vi "remove from memory format.vi"(8 "error in":errorcluster, 10 "CEF_serializable configuration in":refnum<class "CEF_serializable configuration.lvclass">, 11 "memory hierarchy in":T1) -> (0 "error out":errorcluster, 3 "memory hierarchy out":T1)   [LabVIEW 2025, in "CEF.lvlib"]
doc: "Removes an object from an object hierarchy, along with all children.Copyright 2017 National Instruments Corporation\n\nLicensed under the Apache License, Version 2.0 (the \"License\"); you may not use this file except in compliance with the License. You may obtain a copy of the License at http://www.apache.org/licenses/LICENSE-2.0\nUnless required by applicable law or agreed to in writing, software distributed under the License is distributed on an \"AS IS\" BASIS, WITHOUT WARRANTIES OR CONDITIONS OF ANY KIND, either express or implied. See the License for the specific language governing permissions and limitations under the License."
uses:
  CEF.lvlib
  hierarchy repo/memory hierarchy.ctl
  hierarchy repo/full hierarchy.ctl
  hierarchy element.ctl
  serializable configuration/CEF_serializable configuration.lvclass
  serializable configuration/CEF_serializable configuration.lvclass/CEF_serializable configuration.ctl
  <vilib>/Utility/LVClass/Get LV Class Name.vi
  error generator/CEF_error generator.vi
  hierarchy repo/CEF_HierarchyRepo.lvclass
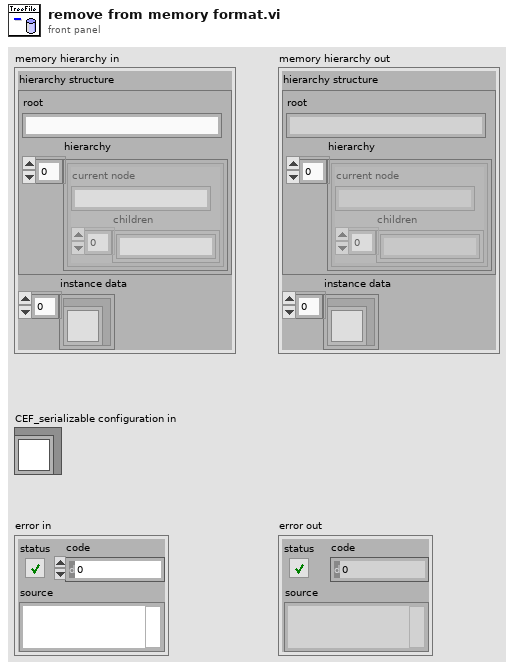
[diagram p1: front panel]
types:
  T1 = typedef "CEF.lvlib/CEF_HierarchyRepo.lvclass/memory hierarchy.ctl" = cluster{"hierarchy structure":T2, "instance data":refnum<class "CEF_serializable configuration.lvclass">[]}
  T2 = typedef "CEF.lvlib/CEF_HierarchyRepo.lvclass/full hierarchy.ctl" = cluster{"root":string, "hierarchy":T3[]}
  T3 = typedef "CEF.lvlib/hierarchy element.ctl" = cluster{"current node":string, "children":string[]}
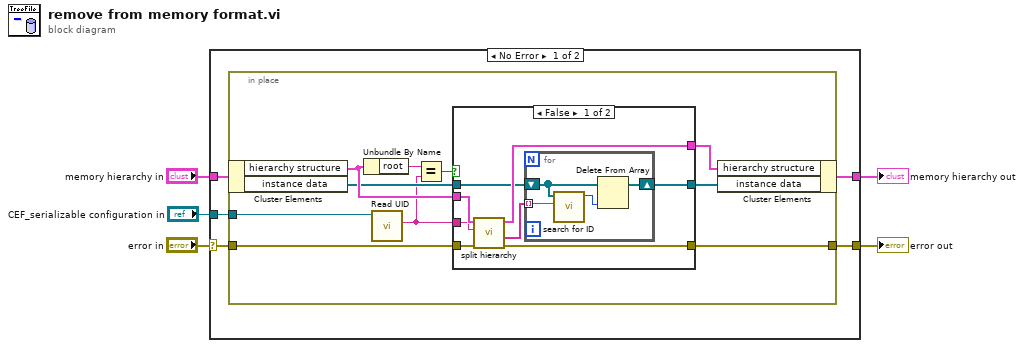
[diagram p0: block diagram]
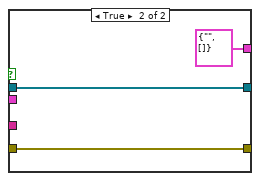
[diagram p2: hidden frame]
diagram:
  n1 = case shown="No Error" "error in" {
    selector: "error in" -> [w7 w37]
    tunnel: [w10 w36] -> w5
    tunnel: "memory hierarchy in" -> [w9 w36]
    tunnel: "CEF_serializable configuration in" -> [w8 _]
    tunnel: [w6 w37] -> w1
    frame No Error {
      n2 = in-place {
        in-place-border: w8 -> [w20]
        in-place-border: w7 -> [w13]
        in-place-border: [w12] -> w6
        n3 = in-place-cluster #1(w9) -> ("hierarchy structure"=w19:T2, "instance data"=w15:refnum<class "CEF_serializable configuration.lvclass">[])
        n4 = Unbundle By Name(w19) -> ("root"=w18:string)
        n5 = call "Read UID.vi"("CEF_Configuration in"=w20) -> ("instance id"=w11:string)  [unwired: 8 in, 2 out]
        n6 = Equal?(x=w18, y=w11) -> (x = y?=w17:bool)
        n7 = case shown="False" w17 {
          tunnel: w19 -> [w28 _]
          tunnel: [w25 T2 {"root"="", "hierarchy"=[]} ("hierarchy structure")] -> w16
          tunnel: w15 -> [w22 w34]
          tunnel: [w21 w34] -> w14
          tunnel: w13 -> [w27 w33]
          tunnel: [w26 w33] -> w12
          tunnel: w11 -> [w24 _]
          frame False {
            n8 = call "split hierarchy.vi"("error in"=w27, "UID to split"=w24, "hierarchy structure"=w28) -> ("error out"=w26:errorcluster, "UIDs moved"=w23:string[], "hierarchy excluding UID"=w25:T2)  [unwired: 5 in, 1 out]
            n9 = for {
              tunnel: w23 -> [w29] mode=indexing
              shift-right: [w31] -> w21
              shift-left: w22 -> [w32]
              n10 = call "search for ID.vi"("instance id"=w29, "instance data"=w32) -> ("index"=w30:i32)  [unwired: 9 in]
              n11 = Delete From Array(array=w32, index=w30) -> (array with subset deleted=w31:refnum<class "CEF_serializable configuration.lvclass">[])  [unwired: 1 in, 1 out]
            }
          }
          frame True {
          }
        }
        n12 = in-place-cluster #1("hierarchy structure"=w16, "instance data"=w14) -> (w10:T1)
      }
    }
    frame Error {
    }
  }
  "memory hierarchy out" <- w5
  "error out" <- w1
